vi "325-340 log(SubVI).vi"(11 "Instrument":T2={"325 Resource "="GPIB0::13::INSTR", "Input (0:A) 325"=0, "Heater Output (1:1) 325"=1, "340 Resource"="GPIB0::14::INSTR", "Input (0:A) 340"=0, "Loop (0: 1)"=0, "Input (0:B) 340"=1, "Loop (1: 1)"=2, "340 Status"=refnum, "Instrument Type"=enum."PPMS", "quantum design"=refnum, "semaphore 325"=refnum, "TCP master instance"=refnum, "M24C Resource"="GPIB0::24::INSTR", "4G supply"="GPIB0::24::INSTR", "Temp Status 24C"=refnum, "Temp"=refnum, "9T信号"=refnum, "limit"={"Field limit"=0.0, "Field rate limit"=0.0, "Temp limit"=0.0, "Temp low limit"=0.0, "Temp rate limit "=0.0}, "4g supply status"=refnum, "vi路径"="", "in-plane"="", "out-plane"="", "in-plane signal"=FALSE, "out-plane signal"=FALSE, "in plane 信号"=refnum, "pzt volt"=refnum, "Aborting"=refnum, "数据文件"=refnum, "warning"=refnum, "750 visa"="", "750 rotate"="", "335 Status 2"=refnum, "335 Resource "="GPIB0::24::INSTR", "Input (0:A) 335"=0, "Input (0:B) 335"=1, "Heater Output (1:1) 335"=1, "semaphore 340"=refnum, "semaphore 335"=refnum, "325 Status"=refnum} {"Loop (1: 1)" items=["1"=1, "2"=2]; "Loop (0: 1)" items=["1"=1, "2"=2]; "Input (0:B) 340" items=["A", "B", "C", "D"]; "Heater Output (1:1) 335" items=["1"=1, "2"=2]; "Input (0:B) 335" items=["A", "B"]; "Input (0:A) 335" items=["A", "B"]; "Heater Output (1:1) 325" items=["1"=1, "2"=2]; "Input (0:A) 325" items=["A", "B"]; "Input (0:A) 340" items=["1"=1, "2"=2]}) -> (3 "output cluster":T1)   [LabVIEW 2019, in "Get value.lvlib"]
uses:
  Get value.lvlib
  ctl/Instrument.ctl
  <vilib>/NI/Modbus Library/API/Master/Modbus Master.lvclass
  ctl/335 state.ctl
  ctl/Instrument Type.ctl
  C:/Users/whmfc/Desktop/MEASURE/lib/QDInstrument.dll
  lib/QDInstrument.dll
  ctl/limit.ctl
  ctl/9T mag field stauts.ctl
  ctl/warning.ctl
  lib/Lake Shore 325/Lake Shore 325.lvlib
  lib/Lake Shore 340/Lake Shore Cryotronics 340.lvlib
panel:
  out "error out":errorcluster
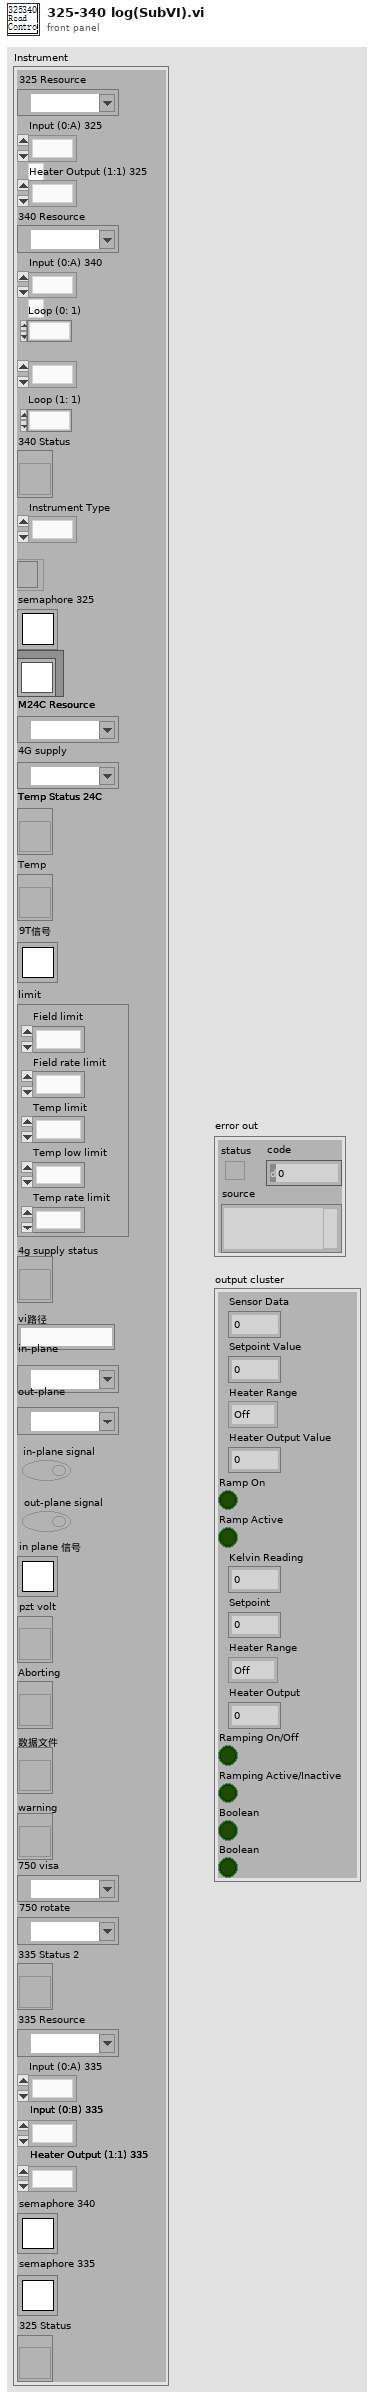
[diagram p1: front panel]
types:
  T1 = cluster{"Sensor Data":dbl, "Setpoint Value":dbl, "Heater Range":enum16{"Off", "Low", "High"}, "Heater Output Value":dbl, "Ramp On":bool, "Ramp Active":bool, "Kelvin Reading":dbl, "Setpoint":dbl, "Heater Range":enum16{"Off", "1", "2", "3", "4", "5"}, "Heater Output":dbl, "Ramping On/Off":bool, "Ramping Active/Inactive":bool, "Boolean":bool, "Boolean":bool}
  T2 = typedef "Instrument.ctl" = cluster{"325 Resource ":refnum<visa-resource-name>, "Input (0:A) 325":u16, "Heater Output (1:1) 325":u16, "340 Resource":refnum<visa-resource-name>, "Input (0:A) 340":u16, "Loop (0: 1)":u16, "Input (0:B) 340":u16, "Loop (1: 1)":u16, "340 Status":refnum<vi>, "Instrument Type":T3, "quantum design":refnum<k24>, "semaphore 325":T4, "TCP master instance":refnum<class "Modbus Master.lvclass">, "M24C Resource":refnum<visa-resource-name>, "4G supply":refnum<visa-resource-name>, "Temp Status 24C":refnum<vi>, "Temp":refnum<vi>, "9T信号":T4, "limit":T5, "4g supply status":refnum<vi>, "vi路径":string, "in-plane":refnum<visa-resource-name>, "out-plane":refnum<visa-resource-name>, "in-plane signal":bool, "out-plane signal":bool, "in plane 信号":T4, "pzt volt":refnum<vi>, "Aborting":refnum<vi>, "数据文件":refnum<vi>, "warning":refnum<vi>, "750 visa":refnum<visa-resource-name>, "750 rotate":refnum<visa-resource-name>, "335 Status 2":refnum<vi>, "335 Resource ":refnum<visa-resource-name>, "Input (0:A) 335":u16, "Input (0:B) 335":u16, "Heater Output (1:1) 335":u16, "semaphore 340":T4, "semaphore 335":T4, "325 Status":refnum<vi>}
  T3 = typedef "Instrument Type.ctl" = enum16{"PPMS", "VersaLab", "DynaCool", "SVSM", "PPMS-Rotate", "Lakeshore335", "lengtou2", "9T mag", "9T cmag rotate", "test"}
  T4 = typedef "Semaphore RefNum" = refnum<k1>
  T5 = typedef "limit.ctl" = cluster{"Field limit":dbl, "Field rate limit":dbl, "Temp limit":dbl, "Temp low limit":dbl, "Temp rate limit ":dbl}
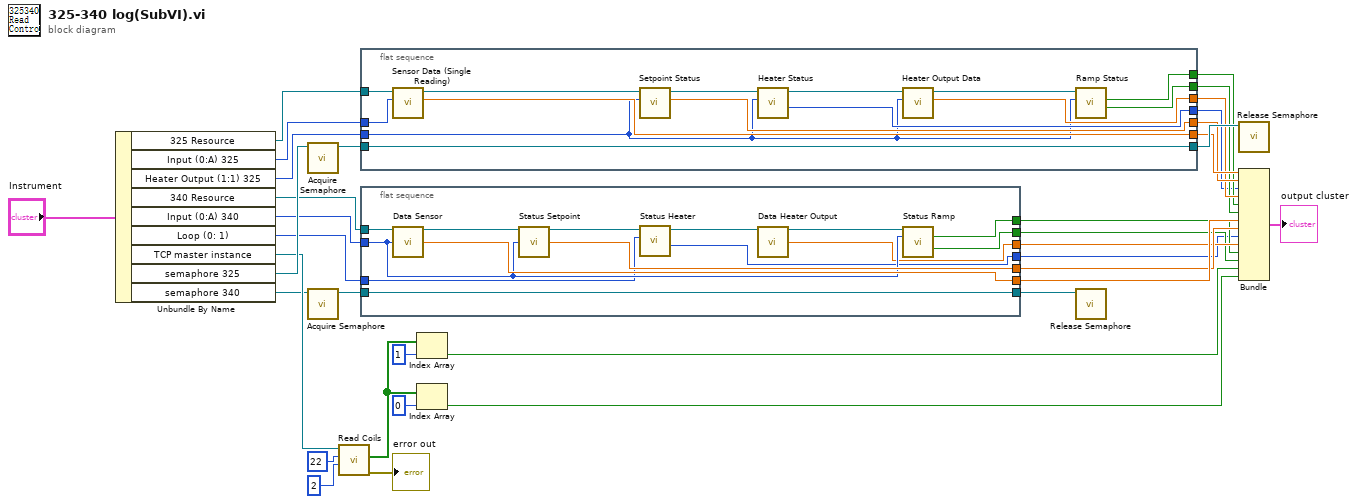
[diagram p0: block diagram]
diagram:
  n1 = Unbundle By Name("Instrument") -> ("325 Resource"=w22:refnum<visa-resource-name>, "Input (0:A) 325"=w21:u16, "Heater Output (1:1) 325"=w26:u16, "340 Resource"=w16:refnum<visa-resource-name>, "Input (0:A) 340"=w15:u16, "Loop (0: 1)"=w11:u16, "TCP master instance"=w19:refnum<class "Modbus Master.lvclass">, "semaphore 325"=w20:T4, "semaphore 340"=w12:T4)
  n2 = call <vilib>:"Acquire Semaphore.vi"("semaphore"=w20) -> ("semaphore out"=w29:T4)  [unwired: 4 in, 2 out]
  n3 = call <vilib>:"Acquire Semaphore.vi"("semaphore"=w12) -> ("semaphore out"=w14:T4)  [unwired: 4 in, 2 out]
  n4 = call-dynamic "Read Coils.vi"("number of inputs"=u16 2, "starting address"=u16 22, "Modbus master in"=w19) -> ("error out"=→"error out":errorcluster, "coils"=w35:bool[])  [unwired: 6 in, 1 out]
  n5 = flat-sequence {
    tunnel: w29 -> [w49]
    tunnel: [w49] -> w30
    tunnel: [w42] -> w17
    tunnel: w26 -> [w36]
    tunnel: w21 -> [w37]
    tunnel: w22 -> [w43]
    tunnel: [w46] -> w24
    tunnel: [w45] -> w1
    tunnel: [w44] -> w23
    tunnel: [w41] -> w25
    tunnel: [w38] -> w18
    frame #0 {
      n6 = call "Sensor Data (Single Reading).vi"("Sensor Input (0:A)"=w37, "VISA resource name"=w43) -> ("Sensor Data"=w41:dbl, "VISA resource name out"=w40:refnum<visa-resource-name>)  [unwired: 7 in, 1 out]
      n7 = call "Setpoint Status.vi"("Loop (1:Loop 1)"=w36, "VISA resource name"=w40) -> ("Setpoint Value"=w46:dbl, "VISA resource name out"=w48:refnum<visa-resource-name>)  [unwired: 7 in, 1 out]
      n8 = call "Heater Status.vi"("Loop (1:Loop 1)"=w36, "VISA resource name"=w48) -> ("Heater Range"=w45:enum16{"Off", "Low", "High"}, "VISA resource name out"=w47:refnum<visa-resource-name>)  [unwired: 7 in, 1 out]
      n9 = call "Heater Output Data.vi"("Loop (1:Loop 1)"=w36, "VISA resource name"=w47) -> ("Heater Output Value"=w44:dbl, "VISA resource name out"=w39:refnum<visa-resource-name>)  [unwired: 7 in, 1 out]
      n10 = call "Ramp Status.vi"("Loop (1:Loop 1)"=w36, "VISA resource name"=w39) -> ("Ramp Active"=w42:bool, "Ramp On"=w38:bool)  [unwired: 5 in, 3 out]
    }
  }
  n11 = flat-sequence {
    tunnel: [w61] -> w9
    tunnel: w16 -> [w63]
    tunnel: w15 -> [w59]
    tunnel: [w62] -> w4
    tunnel: [w60] -> w10
    tunnel: [w57] -> w5
    tunnel: [w54] -> w8
    tunnel: [w55] -> w13
    tunnel: w14 -> [w55]
    tunnel: w11 -> [w51]
    tunnel: [w50] -> w2
    frame #0 {
      n12 = call "Data Sensor.vi"("VISA resource name"=w63, "Input (0: A)"=w59) -> ("VISA resource name out"=w58:refnum<visa-resource-name>, "Kelvin Reading"=w60:dbl)  [unwired: 9 in, 3 out]
      n13 = call "Status Setpoint.vi"("VISA resource name"=w58, "Loop (0: 1)"=w59) -> ("VISA resource name out"=w53:refnum<visa-resource-name>, "Setpoint"=w61:dbl)  [unwired: 11 in, 1 out]
      n14 = call "Status Heater.vi"("Loop"=w51, "VISA resource name"=w53) -> ("Heater Range"=w50:enum16{"Off", "1", "2", "3", "4", "5"}, "VISA resource name out"=w52:refnum<visa-resource-name>)  [unwired: 7 in, 1 out]
      n15 = call "Data Heater Output.vi"("VISA resource name"=w52) -> ("VISA resource name out"=w56:refnum<visa-resource-name>, "Heater Output"=w54:dbl)  [unwired: 12 in, 1 out]
      n16 = call "Status Ramp.vi"("VISA resource name"=w56, "Loop (0: 1)"=w59) -> ("Ramping On/Off"=w57:bool, "Ramping Active/Inactive"=w62:bool)  [unwired: 9 in, 3 out]
    }
  }
  n17 = Index Array(array=w35, index=1) -> (element=w6:bool)
  n18 = Index Array(array=w35, index=0) -> (element=w7:bool)
  n19 = call <vilib>:"Release Semaphore.vi"("semaphore"=w13) -> ()  [unwired: 5 in, 2 out]
  n20 = call <vilib>:"Release Semaphore.vi"("semaphore"=w30) -> ()  [unwired: 5 in, 2 out]
  n21 = Bundle("Sensor Data"=w25, "Setpoint Value"=w24, "Heater Range"=w1, "Heater Output Value"=w23, "Ramp On"=w18, "Ramp Active"=w17, "Kelvin Reading"=w10, "Setpoint"=w9, "Heater Range"=w2, "Heater Output"=w8, "Ramping On/Off"=w5, "Ramping Active/Inactive"=w4, "Boolean"=w6, "Boolean"=w7) -> (→"output cluster":T1)  [unwired: 1 in]
